vi "SetAutomaticParameterMode.vi"(7 "Auto Parameter":T2, 8 "error in (no error)":errorcluster, 10 "Automatic":T1, 11 "Stream in":refnum<class "Stream.lvclass">) -> (0 "error out":errorcluster, 3 "Stream":refnum<class "Stream.lvclass">)   [LabVIEW 2020, in "capture.lvlib" / "Stream.lvclass"]
doc: "SetAutomaticParameterMode."
uses:
  Stream.lvclass
  Camera Automatic Parameters.ctl
  Camera Automatic Parameter Mode.ctl
  Stream.lvclass/Stream.ctl
  common/common.lvlib
  common/bin/gartoolkit_32-1.dll
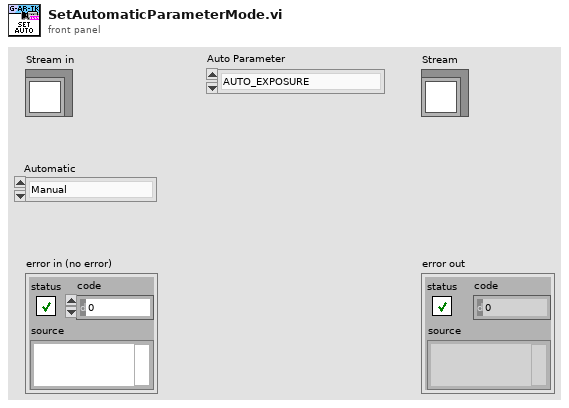
[diagram p1: front panel]
types:
  T1 = typedef "capture.lvlib/Stream.lvclass/Camera Automatic Parameter Mode.ctl" = enum16{"Manual", "Automatic"}
  T2 = typedef "capture.lvlib/Stream.lvclass/Camera Automatic Parameters.ctl" = enum16{"AUTO_EXPOSURE", "AUTO_FOCUS", "AUTO_WHITE_BALANCE", "AUTO_GAIN"}
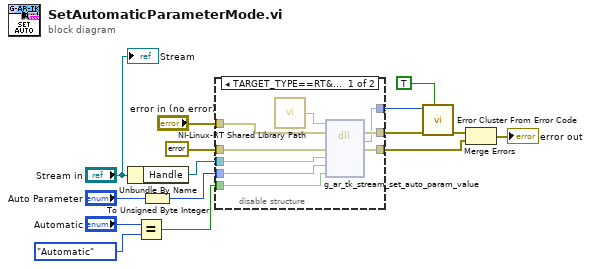
[diagram p0: block diagram]
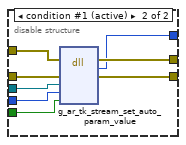
[diagram p2: hidden frame]
diagram:
  n1 = Unbundle By Name("Stream in") -> ("Handle"=w7:refnum<data-value>)
  n2 = Equal?(x="Automatic", y=Camera_Automatic_Parameter_Mode."Automatic") -> (x = y?=w5:bool)
  n3 = To Unsigned Byte Integer(number="Auto Parameter") -> (unsigned 8bit integer=w6:u8)
  n4 = disable-structure shown="TARGET_TYPE==RT&&OS==Linux" {
    disable-tunnel: "error in (no error)" -> [w24 w32]
    disable-tunnel: errorcluster {"status"=FALSE, "code"=0, "source"=""} ("error constant") -> [w23 w31]
    disable-tunnel: w7 -> [w22 w30]
    disable-tunnel: w6 -> [w21 w29]
    disable-tunnel: w5 -> [w20 w28]
    disable-tunnel: [w19 w27] -> w4
    disable-tunnel: [w18 w26] -> w3
    disable-tunnel: [w17 w25] -> w2
    frame condition #0 {
      n5 = call "NI-Linux-RT Shared Library Path.vi"() -> ("Path"=w16:path)
      n6 = dll-call lib="?" fn="g_ar_tk_stream_set_auto_param_value" ("g_ar_toolkit.*.*:g_ar_tk_stream_capture_next")(path in=w16, error in=w24, "error_cluster"=w23, "EDVR_strm"=w22, "parameter"=w21, "automatic"=w20) -> (error out=w19:errorcluster, w18:i32, "error_cluster"=w17:errorcluster)  [unwired: 4 in, 1 out]
    }
    frame condition #1 (active) {
      n7 = dll-call lib="C:/serenial/lib/g-augmented-reality-toolkit/LabVIEW/common/bin/gartoolkit_*-1.*" fn="g_ar_tk_stream_set_auto_param_value" ("g_ar_toolkit.*.*:g_ar_tk_stream_capture_next")(error in=w32, "error_cluster"=w31, "EDVR_strm"=w30, "parameter"=w29, "automatic"=w28) -> (error out=w27:errorcluster, w26:i32, "error_cluster"=w25:errorcluster)  [unwired: 5 in, 1 out]
    }
  }
  n8 = call <vilib>:"Error Cluster From Error Code.vi"("show call chain? (False)"=TRUE, "error in (no error)"=w4, "error code (0)"=w3) -> ("error out"=w12:errorcluster)  [unwired: 6 in]
  n9 = Merge Errors(w12, w2) -> (→"error out":errorcluster)
  "Stream" <- "Stream in"
